vi "Find Length.vi"(10 "Y":dbl[](array[numeric]), 11 "X":dbl[](array[numeric])) -> (0 "Total Length":dbl, 1 "Length Array":dbl[](array[numeric]), 2 "t":dbl[](array[numeric]), 3 "Cumulative Length":dbl[](array[numeric]))   [LabVIEW 2019, in "Tool Path.lvclass"]
uses:
  Tool Path.lvclass
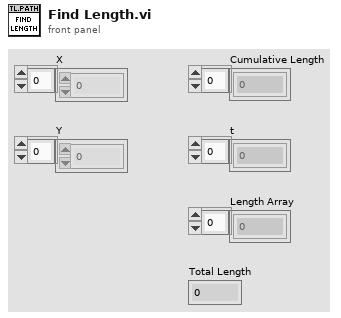
[diagram p1: front panel]
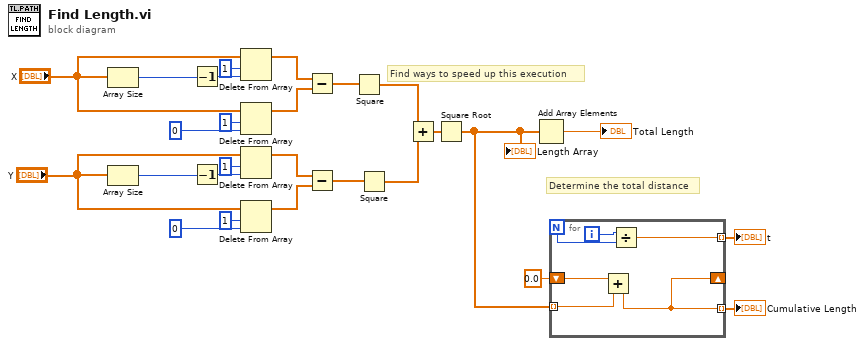
[diagram p0: block diagram]
diagram:
  # "Find ways to speed up this execution"
  # "Determine the total distance"
  n1 = Array Size(array="X") -> (size(s)=w26:i32)
  n2 = Array Size(array="Y") -> (size(s)=w16:i32)
  n3 = Decrement(x=w26) -> (x-1=w25:i32)
  n4 = Decrement(x=w16) -> (x-1=w17:i32)
  n5 = Delete From Array(array="X", length=1, index=w25) -> (array with subset deleted=w13:dbl[])  [unwired: 1 out]
  n6 = Delete From Array(array="X", length=1, index=0) -> (array with subset deleted=w12:dbl[])  [unwired: 1 out]
  n7 = Delete From Array(array="Y", length=1, index=w17) -> (array with subset deleted=w11:dbl[])  [unwired: 1 out]
  n8 = Delete From Array(array="Y", length=1, index=0) -> (array with subset deleted=w10:dbl[])  [unwired: 1 out]
  n9 = Subtract(x=w13, y=w12) -> (x-y=w21:dbl[])
  n10 = Subtract(x=w11, y=w10) -> (x-y=w15:dbl[])
  n11 = Square(x=w21) -> (x^2=w9:dbl[])
  n12 = Square(x=w15) -> (x^2=w8:dbl[])
  n13 = Add(x=w9, y=w8) -> (x+y=w14:dbl[])
  n14 = Square Root(x=w14) -> (sqrt(x)=w7:dbl[])
  "Length Array" <- w7
  n15 = Add Array Elements(numeric array=w7) -> (sum=→"Total Length":dbl)
  n16 = for {
    N -> [w28]
    tunnel: w7 -> [w31] mode=indexing
    shift-right: [w30] -> _
    shift-left: 0.0 -> [w32]
    tunnel: [w30] -> w2 mode=indexing
    tunnel: [w27] -> w1 mode=indexing
    i -> [w29]
    n17 = Add(x=w32, y=w31) -> (x+y=w30:dbl)
    n18 = Divide(x=w29, y=w28) -> (x/y=w27:dbl)
  }
  "Cumulative Length" <- w2
  "t" <- w1
